vi "createEvent.vi"(8 "error in (no error)":errorcluster, 11 "Handler.UserEvent in":refnum<class "Handler.UserEvent.lvclass">) -> (0 "error out":errorcluster, 3 "Handler.UserEvent out":refnum<class "Handler.UserEvent.lvclass">)   [LabVIEW 2017, in "Error Log.lvlib" / "Handler.UserEvent.lvclass"]
uses:
  Handler.UserEvent.lvclass
  Record/Record.lvclass
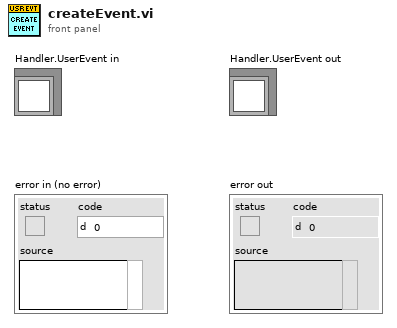
[diagram p1: front panel]
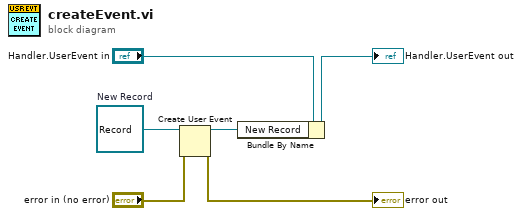
[diagram p0: block diagram]
diagram:
  w5 = refnum<class "Record.lvclass"> refnum  # New Record
  n1 = Create User Event(user event datatype=w5, error in="error in (no error)") -> (user event=w1:refnum<user-event>, error out=→"error out":errorcluster)
  n2 = Bundle By Name(cluster="Handler.UserEvent in", "New Record"=w1) -> (→"Handler.UserEvent out":refnum<class "Handler.UserEvent.lvclass">)
